vi "Transform2d_Times.vi"(9 "Scalar":dbl, 11 "inTRANSFORM":T1={"TRANSLATION"={"X"=0.0, "Y"=0.0}, "ROTATION"={"VALUE"=0.0, "COS"=1.0, "SIN"=0.0}, "xF"=FALSE} {"ROTATION"."SIN" format="%13.4f"; "ROTATION"."COS" format="%13.4f"; "ROTATION"."VALUE" format="%13.4f"; "TRANSLATION"."Y" format="%14.3f"; "TRANSLATION"."X" format="%14.3f"}) -> (3 "TRANSFORM":T1 {"ROTATION"."SIN" format="%13.4f"; "ROTATION"."COS" format="%13.4f"; "ROTATION"."VALUE" format="%13.4f"; "TRANSLATION"."Y" format="%14.3f"; "TRANSLATION"."X" format="%14.3f"})   [LabVIEW 2019, in "Trajectory_Library.lvlib"]
doc: "Scales the transform by the scalar.\n\nParameters:\n - IN TRANSFORM - This TRANSFORM data structure\n - SCALAR - The scalar value to multiply the transform by\n\nResults:\n - OUT TRANSFORM - The multiplied transform data structure"
uses:
  Trajectory_Library.lvlib
  TypeDef/TRANSLATION2D.ctl
  TypeDef/ROTATION2D.ctl
  TypeDef/TRANSFORM2D.ctl
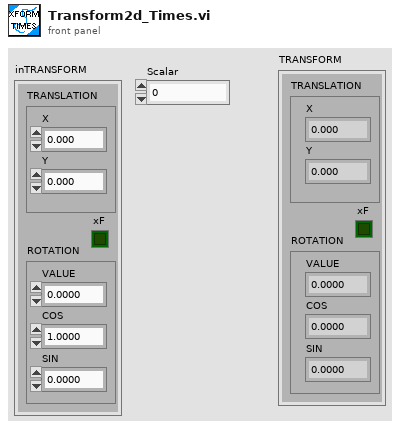
[diagram p1: front panel]
types:
  T1 = typedef "Trajectory_Library.lvlib/TRANSFORM2D.ctl" = cluster{"TRANSLATION":T2, "ROTATION":T3, "xF":bool}
  T2 = typedef "Trajectory_Library.lvlib/TRANSLATION2D.ctl" = cluster{"X":dbl, "Y":dbl}
  T3 = typedef "Trajectory_Library.lvlib/ROTATION2D.ctl" = cluster{"VALUE":dbl, "COS":dbl, "SIN":dbl}
  T4 = typedef "WPILib_Math.lvlib/TRANSLATION2D.ctl" = cluster{"X":dbl, "Y":dbl}
  T5 = typedef "WPILib_Math.lvlib/ROTATION2D.ctl" = cluster{"VALUE":dbl, "COS":dbl, "SIN":dbl}
  T6 = typedef "WPILib_Math.lvlib/TRANSFORM2D.ctl" = cluster{"TRANSLATION":T4, "ROTATION":T5, "xF":bool}
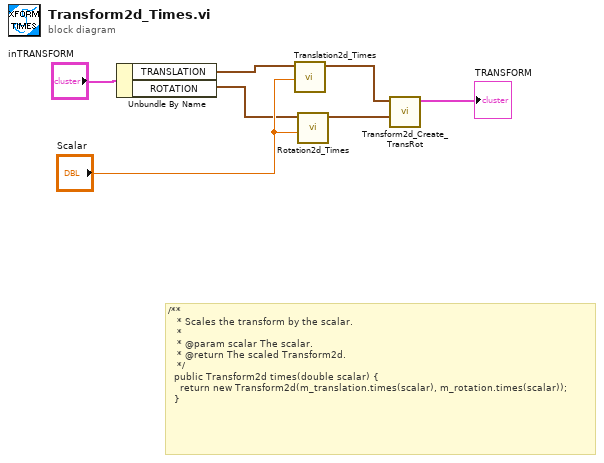
[diagram p0: block diagram]
diagram:
  # "/**\n   * Scales the transform by the scalar.\n   *\n   * @param scalar The scalar.\n   * @return The scaled Transform2d.\n   */\n  public Transform2d times(double scalar) {\n    return new Transform2d(m_translation.times(scalar), m_rotation.times(scalar));\n  }"
  n1 = Unbundle By Name("inTRANSFORM") -> ("TRANSLATION"=w5:T2, "ROTATION"=w2:T3)
  n2 = call "Translation2d_Times.vi"("Scalar"="Scalar", "In Translation"=w5) -> ("Out Translation"=w4:T4)  [unwired: 9 in]
  n3 = call "Rotation2d_Times.vi"("Scalar"="Scalar", "in ROTATION"=w2) -> ("out ROTATION"=w1:T5)  [unwired: 9 in]
  n4 = call "Transform2d_Create_TransRot.vi"("ROTATION"=w1, "TRANSLATION"=w4) -> ("TRANSFORM"=→"TRANSFORM":T6)  [unwired: 9 in]
